vi "make string one-line.vi"(9 "replacement for new line":string=" > ", 11 "multi-line string":string) -> (3 "one-line-string":string)   [LabVIEW 2020]
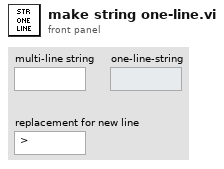
[diagram p1: front panel]
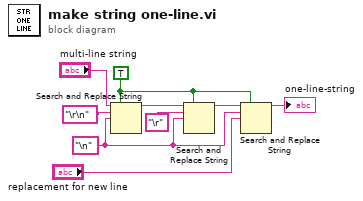
[diagram p0: block diagram]
diagram:
  w8 = "\n" ("search string")
  w6 = TRUE ("replace all? (F)")
  n1 = Search and Replace String(replace all?=w6, input string="multi-line string", search string="\r\n", replace string=w8) -> (result string=w3:string)  [unwired: 4 in, 3 out]
  n2 = Search and Replace String(replace all?=w6, input string=w3, search string="\r", replace string=w8) -> (result string=w7:string)  [unwired: 4 in, 3 out]
  n3 = Search and Replace String(replace all?=w6, input string=w7, search string=w8, replace string="replacement for new line") -> (result string=→"one-line-string":string)  [unwired: 4 in, 3 out]
